vi "SHA3-512 Byte Array Checksum.vi"(11 "buffer":u8[](array[numeric]) format="%02x") -> (3 "digest":string)   [LabVIEW 2020, in "NI_Message Digest API.lvlib"]
doc: "Computes the message digest on a byte array. You must manually select the polymorphic instance you want to use."
uses:
  <vilib>/security/Message Digest/API/NI_Message Digest API.lvlib
  <vilib>/security/Message Digest/SHA-3/NI_SHA-3.lvclass/NI_SHA-3.ctl
  6b0a94b4-5f98-45be-8858-b3dd3cac734b.vi
  6b0a94b4-5f98-45be-8858-b3dd3cac734b.vi/7066ccd8-2cf3-3fe0-00ac-bb816d1ca13f.vi
  <vilib>/security/Message Digest/SHA-3/Get Block Size.vi
  <vilib>/security/Message Digest/SHA-3/Get Block Size.vi/eb1e6525-3e01-40a8-a5c2-e849aaf68d04.vi
  <vilib>/security/Message Digest/SHA-3/Get Block Size.vi/eb1e6525-3e01-40a8-a5c2-e849aaf68d04.vi/00efce51-7697-47ef-971b-245e50795e7f.vi
  <vilib>/security/Message Digest/SHA-3/subVIs/Get Capacity.vi
  <vilib>/security/Message Digest/SHA-3/subVIs/Get Word Type.vi
  <vilib>/security/Message Digest/SHA-3/Reset.vi
  <vilib>/security/Message Digest/SHA-3/Append Block.vi
  <vilib>/security/Message Digest/SHA-3/Pad.vi
  <vilib>/security/Message Digest/SHA-3/Get Digest.vi
  <vilib>/security/Message Digest/SHA-3/NI_SHA-3.lvclass
  <vilib>/Bit Manipulation/NI_Bit Manipulation.lvlib
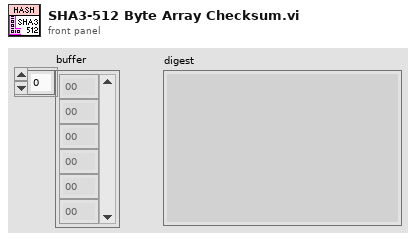
[diagram p1: front panel]
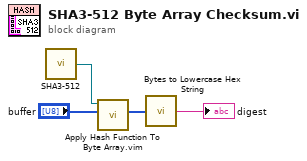
[diagram p0: block diagram]
diagram:
  n1 = call <vilib>:"SHA3-512.vi"() -> ("Hash Function out"=w3:refnum<class "NI_SHA-3.lvclass">)
  n2 = call "Apply Hash Function To Byte Array.vim"("buffer"="buffer", "Hash Function in (SHA-256)"=w3) -> ("digest"=w1:u8[])  [unwired: 8 in, 1 out]
  n3 = call <vilib>:"Bytes to Lowercase Hex String.vi"("bytes"=w1) -> ("hex string"=→"digest":string)
